vi "test.vi"() -> ()   [LabVIEW 2017]
panel:
  in  "Speed_R":dbl
  in  "speed_L":dbl
  in  "dir":bool
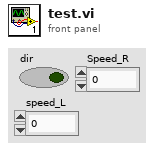
[diagram p1: front panel]
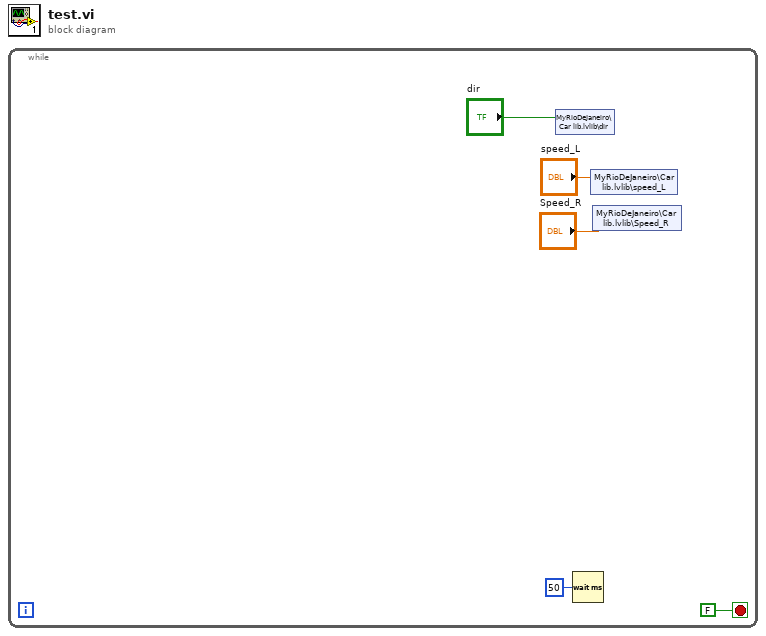
[diagram p0: block diagram]
diagram:
  n1 = while {
    stop <- FALSE stop-if-true
    n2 = shared-variable "MyRioDeJaneiro\\Car lib.lvlib\\dir"("dir") -> ()  [unwired: 1 in, 1 out]
    n3 = Wait (ms)(milliseconds to wait=u32 50) -> ()  [unwired: 1 out]
    n4 = shared-variable "MyRioDeJaneiro\\Car lib.lvlib\\speed_L"("speed_L") -> ()  [unwired: 1 in, 1 out]
    n5 = shared-variable "MyRioDeJaneiro\\Car lib.lvlib\\Speed_R"("Speed_R") -> ()  [unwired: 1 in, 1 out]
  }
